vi "niRFUtil RFHS CONV VoltSquare to dBm (real array).vi"(0 "Real Array (Volt Square)":T1 min=0 max=127 format="%.2f", 1 "Signal Type: Complex (F)/ Real (T)":bool, 5 "Impedence (ohm)":sgl=50.0 format="%.2g", 11 "error in (no error)":errorcluster) -> (4 "Real Array (dBm)":T1 min=0 max=127 format="%.2f", 15 "error out":errorcluster)   [LabVIEW 2015, in "niRFUtil.lvlib"]
uses:
  niRFUtil.lvlib
  Includes/niRFUtil INC Real Array.ctl
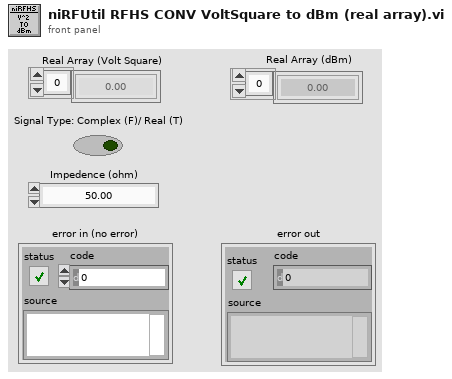
[diagram p1: front panel]
types:
  T1 = typedef "niRFUtil.lvlib/niRFUtil INC Real Array.ctl" = sgl[]
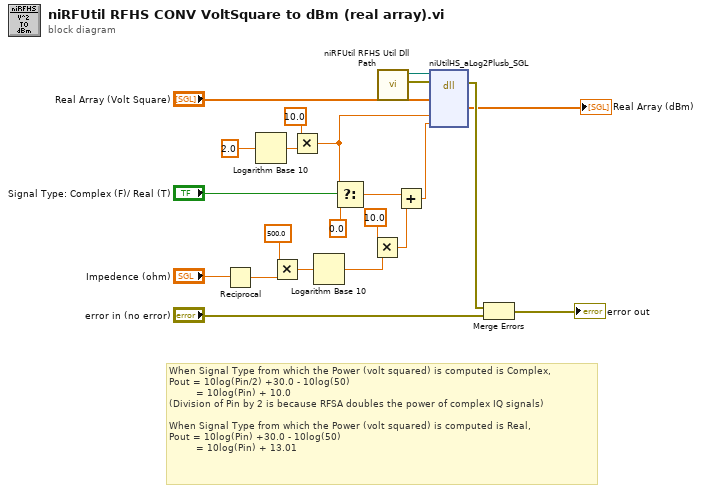
[diagram p0: block diagram]
diagram:
  # "When Signal Type from which the Power (volt squared) is computed is Complex, \nPout = 10log(Pin/2) +30.0 - 10log(50)\n         = 10log(Pin) + 10.0\n(Division of Pin by 2 is because RFSA doubles the power of complex IQ signals)\n\nWhen Signal Type from which the Power (volt squared) is computed is Real, \nPout = 10log(Pin) +30.0 - 10log(50)\n         = 10log(Pin) + 13.01"
  n1 = Reciprocal(x="Impedence (ohm)") -> (1/x=w10:sgl)
  n2 = Logarithm Base 10(1:sgl 2.0 ("x")) -> (0:w17:sgl)
  n3 = Multiply(x=sgl 500.0, y=w10) -> (x*y=w11:sgl)
  n4 = Multiply(x=sgl 10.0, y=w17) -> (x*y=w5:sgl)
  n5 = Logarithm Base 10(1:w11) -> (0:w13:sgl)
  n6 = Select(t=w5, s="Signal Type: Complex (F)/ Real (T)", f=sgl 0.0 ("t")) -> (s? t:f=w7:sgl)
  n7 = Multiply(x=sgl 10.0, y=w13) -> (x*y=w8:sgl)
  n8 = call "niRFUtil RFHS Util Dll Path.vi"() -> ("error out"=w15:errorcluster, "Path"=w16:path)  [unwired: 7 in, 3 out]
  n9 = Add(x=w7, y=w8) -> (x+y=w4:sgl)
  n10 = dll-call lib="M:/RfProtocols/RFmx/DLLs/niRFHS/trunk/2.1/dist/win32U/niRFHS_avx.dll" fn="niUtilHS_aLog2Plusb_SGL" label="a*log2(x/2)+a+b"(path in=w16, error in=w15, "iBuf"="Real Array (Volt Square)", "a"=w5, "b"=w4) -> (error out=w14:errorcluster, "oBuf"=→"Real Array (dBm)":sgl[])  [unwired: 6 in, 1 out]
  n11 = Merge Errors(w14, "error in (no error)") -> (→"error out":errorcluster)
